vi "Take_C1_C2_Then_C1+C2.vi"(3 "Mode":T5, 5 "Traverse line In":T2 {"Row Duration (mins)" format="%#.1f"; "Row No" min=0; "Trace Gas Concentration (%)" min=0.0 format="%#.2f"; "Emission Rate (l/min)" format="%#.2f"; "Tunnel Speed" format="%#.2f"; "Start X" format="%#.2f"; "Start Y" format="%#.2f"; "Start Z" format="%#.2f"; "End X" format="%#.2f"; "End Y" format="%#.2f"; "End Z" format="%#.2f"; "Averaging time (min)" min=0.0 format="%#.1f"}) -> (0 "Error Message":string, 1 "Status":T1, 2 "Traverse line Out":T2 {"Row Duration (mins)" format="%#.1f"; "Row No" min=0; "Trace Gas Concentration (%)" min=0.0 format="%#.2f"; "Emission Rate (l/min)" format="%#.2f"; "Tunnel Speed" format="%#.2f"; "Start X" format="%#.2f"; "Start Y" format="%#.2f"; "Start Z" format="%#.2f"; "End X" format="%#.2f"; "End Y" format="%#.2f"; "End Z" format="%#.2f"; "Averaging time (min)" min=0.0 format="%#.1f"})   [LabVIEW 2010]
uses:
  Gen Trav/Traverse_cluster.ctl
  Gen Trav/Spacing.ctl
  Controls/Multi_run_mode.ctl
  Controls/User_Specific_mode.ctl
  Gen Trav/Multi_Run_Status.ctl
  Controls/Save_Data.ctl
  Controls/Setup.ctl
  Plug in sub vis/Extra_info.vi
  Globals/Meas_global.vi
panel:
  out "UA/Q 2":dbl
  out "UA/Q":dbl
  out "Source1 Ref?":bool
  out "Reference Position":dbl
  out "XY Graph":cluster{dbl[], dbl[]}(graph)
  out "Ch Values":string[](array[string])
  out "Ch Names":string[](array[string])
  # "X           Y            Z"
  # "Start"
  # "End"
  # "X           Y            Z"
  # "Start"
  # "End"
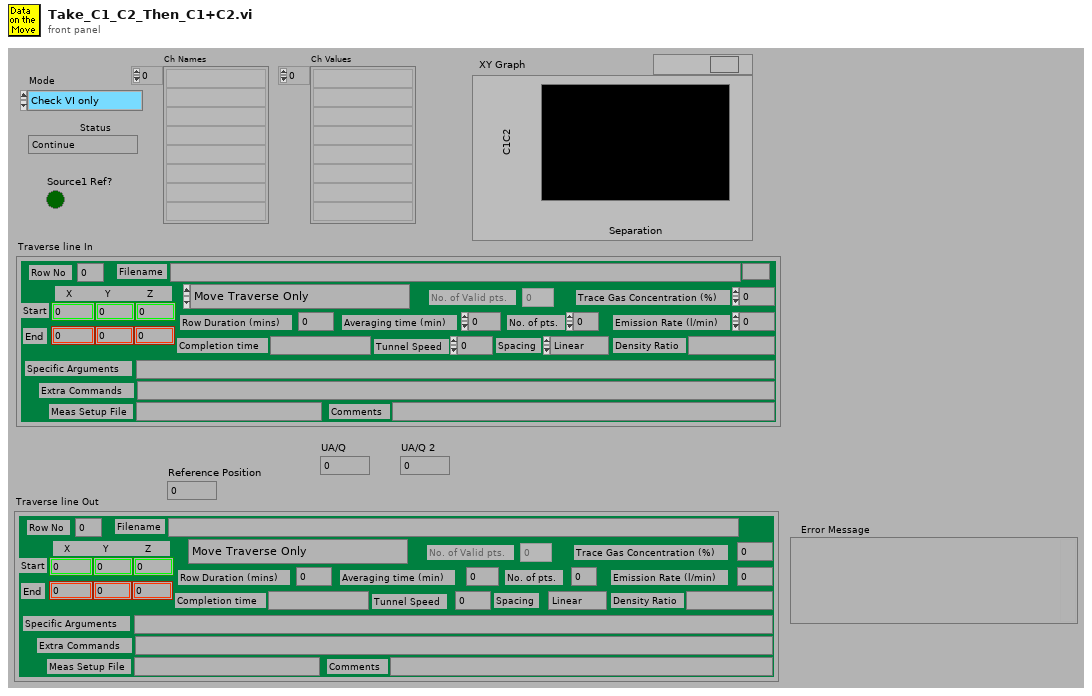
[diagram p1: front panel]
types:
  T1 = typedef "Multi_Run_Status.ctl" = enum16{"Continue", "Jump to Next Point", "Jump to Next Row", "Jump To Fall Back", "Terminate Run"}
  T2 = typedef "Traverse_cluster.ctl" = cluster{"Start X":dbl, "Start Y":dbl, "Start Z":dbl, "End X":dbl, "End Y":dbl, "End Z":dbl, "No. of pts.":i32, "Spacing":T3, "Filename":path, "Tunnel Speed":dbl, "Averaging time (min)":dbl, "Extra Commands":string, "Specific Arguments":string, "Emission Rate (l/min)":dbl, "Trace Gas Concentration (%)":dbl, "Density Ratio":string, "Comments":string, "Row No":i32, "Row Type Selector":T4, "Completion time":string, "Row Duration (mins)":dbl, "No. of Valid pts.":i32, "Meas Setup File":string}
  T3 = typedef "Spacing.ctl" = enum16{"Linear", "Log", "Gauss", "Specified", "N/A"}
  T4 = typedef "Multi_run_mode.ctl" = enum16{"Move Traverse Only", "Set Tunnel Speed Only", "Set Source Only", "Set Measurement Conditions", "Single Measurement", "Vertical Profile", "Lateral Profile", "Longitudinal Profile", "Explore Volume", "Multi-Axis Profile", "Auto Calibrate", "Meas Fast FID Bkgnd", "Check Beam Power", "Scanning Valve Measurement", "Run VI Named:", "Set ADAM Ch", "Wait (minutes)", "Send Message", "Synchronize With:", "Fall Back to this Row", "Turn Off Row Repeating", "Blank Row"}
  T5 = typedef "User_Specific_mode.ctl" = enum16{"Check VI only", "Run VI"}
  T6 = enum16{"Source 1 only", "Source 2 only", "Both Sources"}
  T7 = typedef "Save_Data.ctl" = enum16{"Save No Data", "Save Data"}
  T8 = typedef "Setup.ctl" = enum16{"Run Program", "Show Setup", "Save Current Setup", "Setup Front Panel"}
  T9 = typedef "Status_Cluster.ctl" = cluster{"Status":T1, "Error Type":string, "Error Description":string}
  T10 = typedef "Velocity_cluster.ctl" = cluster{"Name":string, "U":dbl, "u^2":dbl, "u^3/(u^2)^(1.5)":dbl, "u^4/(u^2)^2 -3":dbl, "% u'/U":dbl, "Mean % Err":dbl, "u^4":dbl}
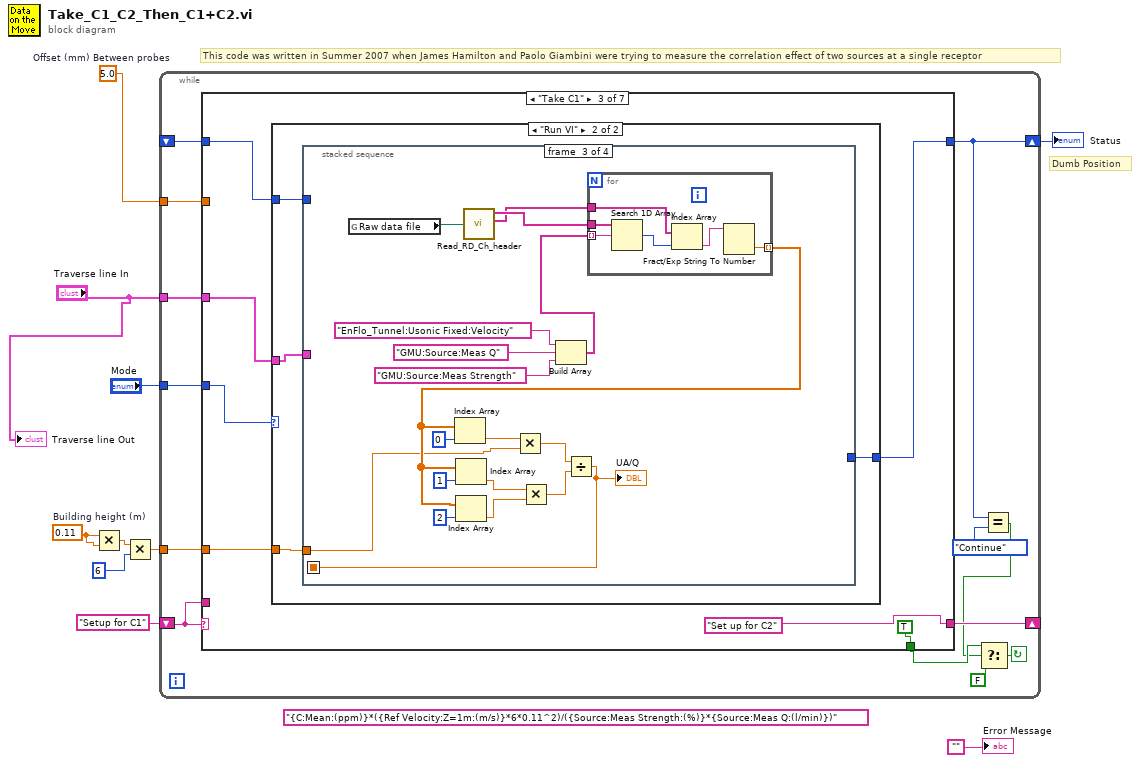
[diagram p0: block diagram]
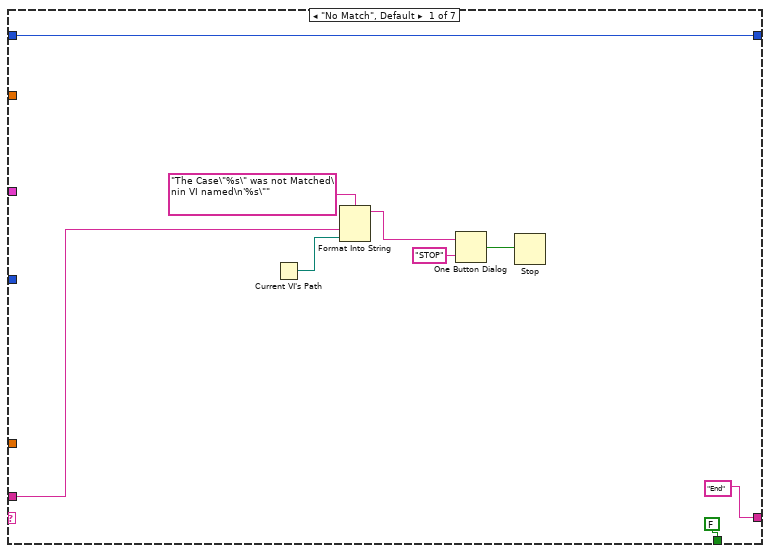
[diagram p2: hidden frame]
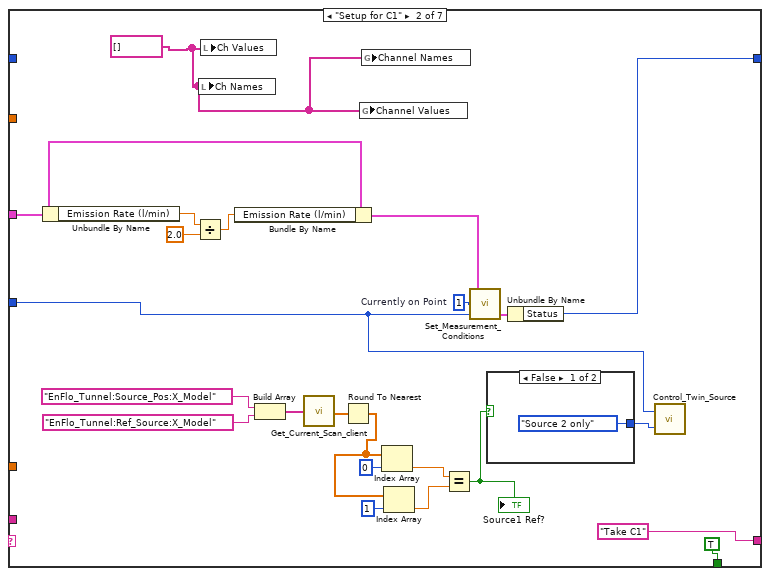
[diagram p3: hidden frame]
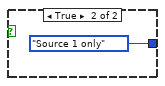
[diagram p4: hidden frame]
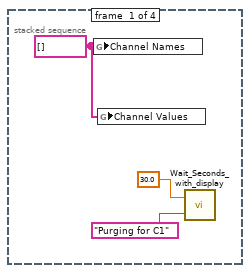
[diagram p6: hidden frame]
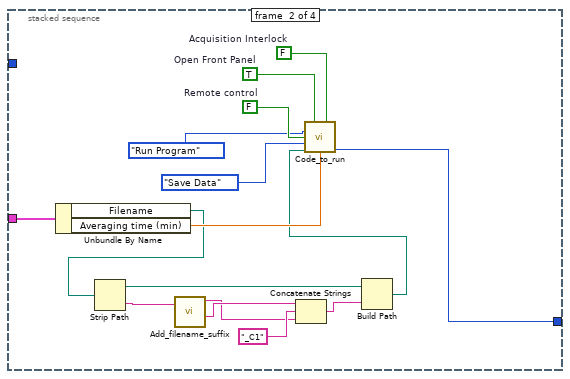
[diagram p7: hidden frame]
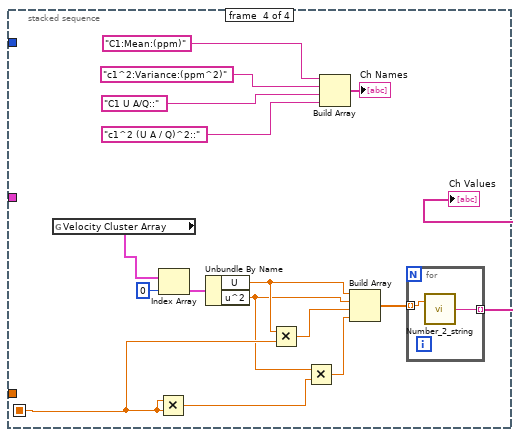
[diagram p8: hidden frame]
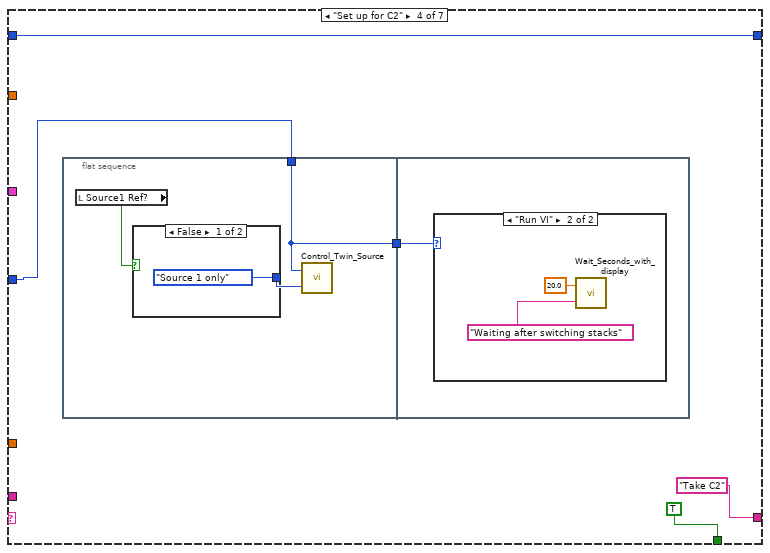
[diagram p9: hidden frame]
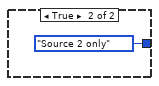
[diagram p10: hidden frame]
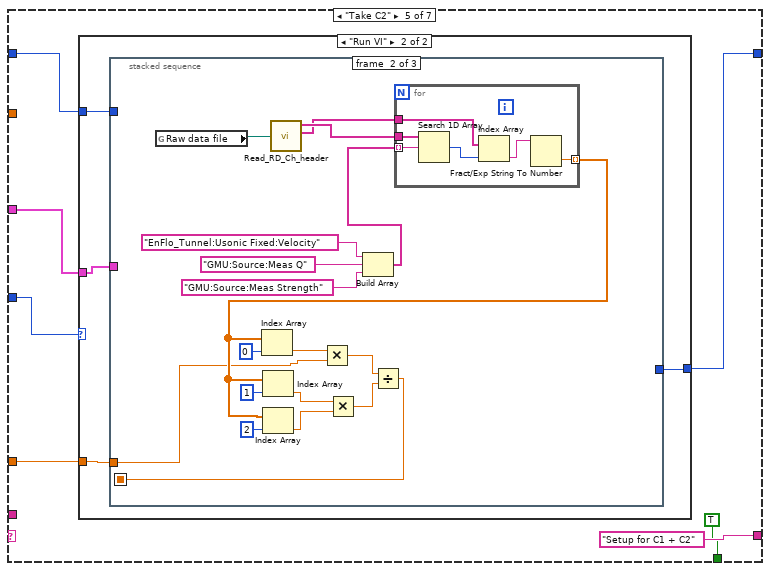
[diagram p12: hidden frame]
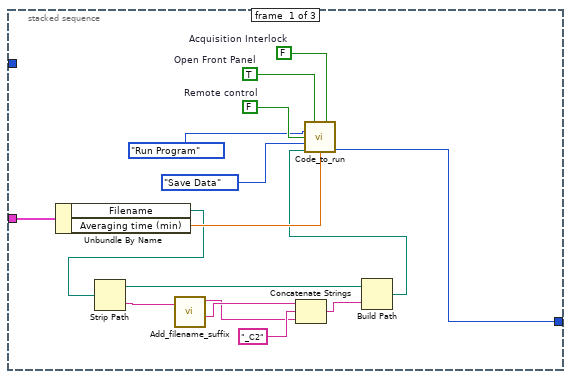
[diagram p14: hidden frame]
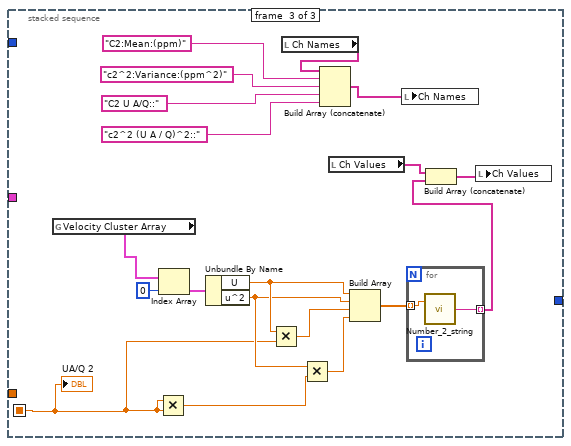
[diagram p15: hidden frame]
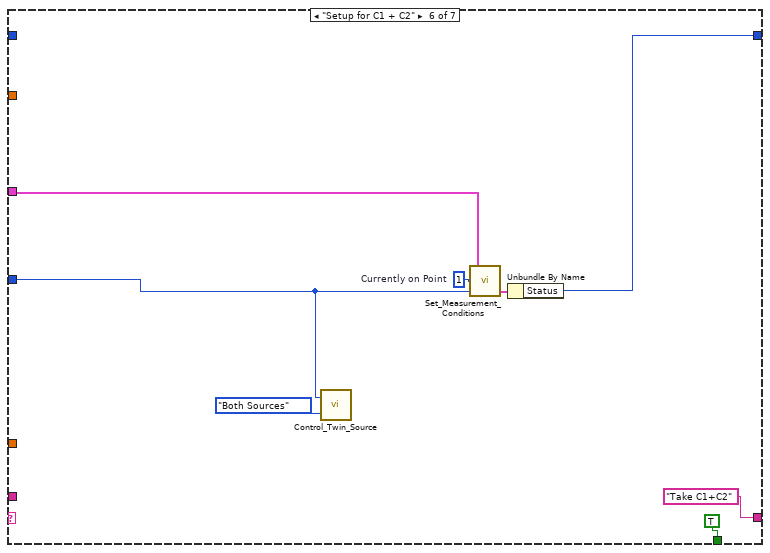
[diagram p16: hidden frame]
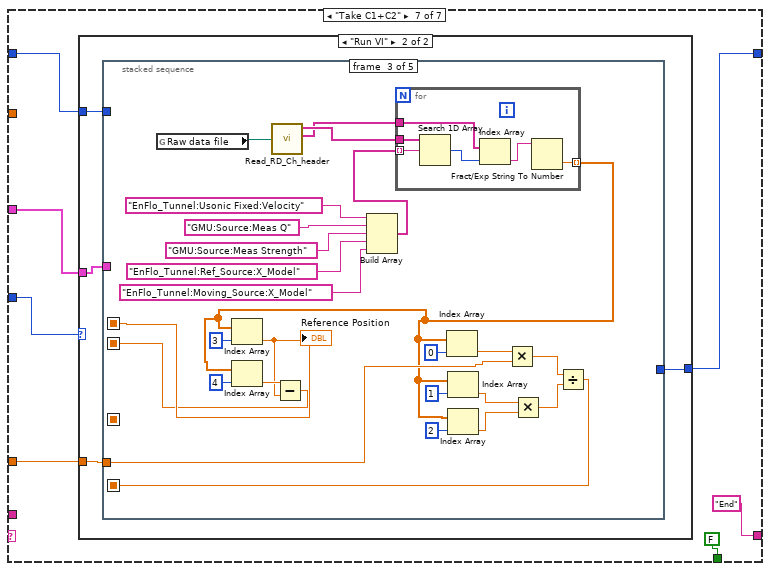
[diagram p17: hidden frame]
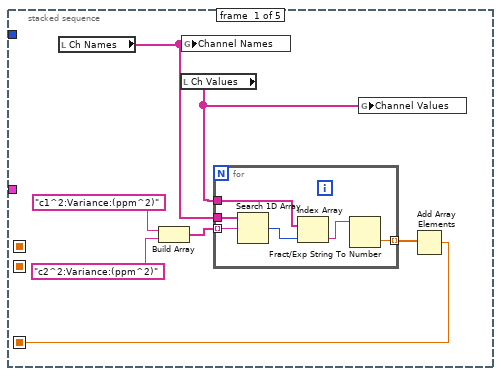
[diagram p19: hidden frame]
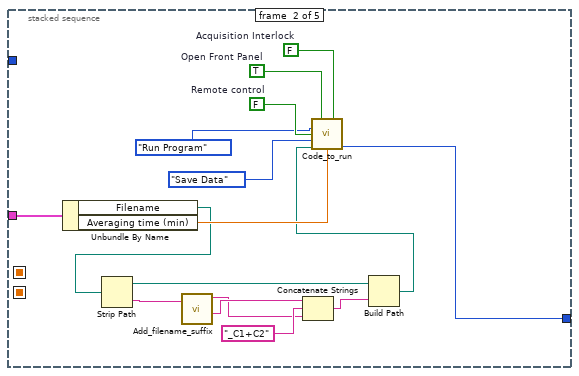
[diagram p20: hidden frame]
diagram:
  w5 = 0.11  # Building height (m)
  (unwired) "{C:Mean:(ppm)}*({Ref Velocity:Z=1m:(m/s)}*6*0.11^2)/({Source:Meas Strength:(%)}*{Source:Meas Q:(l/min)})"
  w7 = 5.0  # Offset (mm) Between probes
  # "This code was written in Summer 2007 when James Hamilton and Paolo Giambini were trying to measure the correlation effect of two sources at a single receptor"
  # "Dumb Position"
  n1 = Multiply(x=w5, y=w5) -> (x*y=w4:dbl)
  n2 = Multiply(x=w4, y=6) -> (x*y=w2:dbl)
  n3 = while {
    shift-left: _ -> [w20]
    shift-right: [w15] -> w8
    tunnel: "Traverse line In" -> [w22]
    tunnel: "Mode" -> [w23]
    shift-left: "Setup for C1" -> [w21]
    shift-right: [w19] -> _
    tunnel: w7 -> [w12]
    tunnel: w2 -> [w11]
    stop <- w13 continue-if-true
    n4 = case shown="\"Take C1\"" w21 {
      tunnel: w22 -> [_ w53 w63 _ w149 w221 w230]
      tunnel: w23 -> [_ w36 w64 w132 w150 w217 w231]
      tunnel: [FALSE ("Update Datum Powers?") TRUE ("Update Datum Powers?") TRUE ("Update Datum Powers?") TRUE ("Update Datum Powers?") TRUE ("Update Datum Powers?") TRUE ("Update Datum Powers?") FALSE ("Update Datum Powers?")] -> w18
      tunnel: ["End" "Take C1" "Set up for C2" "Take C2" "Setup for C1 + C2" "Take C1+C2" "End"] -> w19
      tunnel: w21 -> [w25 _ _ _ _ _ _]
      tunnel: w20 -> [w24 _ w61 w135 w147 _ w228]
      tunnel: [w24 w48 w58 w135 w144 w219 w225] -> w15
      tunnel: w12 -> [_ _ _ _ _ _ _]
      tunnel: w11 -> [_ _ w62 _ w148 _ w229]
      frame "No Match", Default {
        n5 = Current VI's Path() -> (path=w28:path)
        n6 = Format Into String(format string="The Case\"%s\" was not Matched\nin VI named\n'%s\"" ("Format String"), w25, w28) -> (resulting string=w31:string)  [unwired: 2 in, 1 out]
        n7 = One Button Dialog(message=w31, button name ("OK")="STOP") -> (true=w29:bool)
        n8 = Stop(stop? (T)=w29) -> ()
      }
      frame "Setup for C1" {
        w35 = string[] [] ("Ch Values")
        w54 = 1  # Currently on Point
        n9 = Unbundle By Name(w53) -> ("Emission Rate (l/min)"=w52:dbl)
        n10 = Divide(x=w52, y=2.0) -> (x/y=w50:dbl)
        n11 = local write "Ch Names"(w35) -> ()
        n12 = local write "Ch Values"(w35) -> ()
        n13 = Bundle By Name(cluster=w53, "Emission Rate (l/min)"=w50) -> (w49:T2)
        n14 = Build Array("EnFlo_Tunnel:Source_Pos:X_Model", "EnFlo_Tunnel:Ref_Source:X_Model" ("Channel Name")) -> (w43:string[])
        n15 = call "Get_Current_Scan_client.vi"("ADAM Ch Names"=w43) -> ("Numerical Values"=w34:dbl[])  [unwired: 3 out]
        n16 = Round To Nearest(number=w34) -> (nearest integer value=w33:dbl[])
        n17 = global write "Extra_info.vi" "Channel Values"(w35) -> ()
        n18 = global write "Extra_info.vi" "Channel Names"(w35) -> ()
        n19 = Index Array(array=w33, index=0) -> (element=w39:dbl)
        n20 = Index Array(array=w33, index=1) -> (element=w40:dbl)
        n21 = Equal?(x=w39, y=w40) -> (x = y?=w38:bool)
        "Source1 Ref?" <- w38
        n22 = call "Set_Measurement_Conditions.vi"("Simulate/Run"=w36, "Currently on Point"=w54, "Traverse line"=w49) -> ("Status Cluster"=w55:T9)  [unwired: 2 out]
        n23 = case shown="False" w38 {
          tunnel: [T6."Source 2 only" ("Mode") T6."Source 1 only" ("Mode")] -> w37
          frame False {
          }
          frame True {
          }
        }
        n24 = Unbundle By Name(w55) -> ("Status"=w48:T1)
        n25 = call "Control_Twin_Source.vi"("Control"=w37, "Mode"=w36) -> ()
      }
      frame "Take C1" {
        n26 = case shown="\"Run VI\"" w64 {
          tunnel: [w65 w69] -> w58
          tunnel: w63 -> [_ w68]
          tunnel: w62 -> [_ w67]
          tunnel: w61 -> [w65 w66]
          frame "Check VI only" {
          }
          frame "Run VI" {
            n27 = stacked-sequence {
              seq-local: [_ _ w89 _] -> [_ _ _ w119]
              tunnel: [_ w88 _ _] -> w69
              tunnel: w68 -> [_ w87 _ _]
              tunnel: w67 -> [_ _ w94 _]
              tunnel: w66 -> [_ _ _ _]
              frame #0 {
                w72 = string[] [] ("Channel Names")
                n28 = global write "Extra_info.vi" "Channel Names"(w72) -> ()
                n29 = global write "Extra_info.vi" "Channel Values"(w72) -> ()
                n30 = call "Wait_Seconds_with_display.vi"("Message"="Purging for C1", "Seconds to wait"=30.0) -> ()  [unwired: 2 out]
              }
              frame #1 {
                w83 = FALSE  # Acquisition Interlock
                w84 = TRUE  # Open Front Panel
                w86 = FALSE  # Remote control
                n31 = Unbundle By Name(w87) -> ("Filename"=w74:path, "Averaging time (min)"=w85:dbl)
                n32 = Strip Path(path=w74) -> (stripped path=w75:path, name=w80:string)
                n33 = call "Add_filename_suffix.vi"("Filename"=w80) -> ("Original Suffix"=w77:string, "Base name"=w79:string)  [unwired: 1 in, 2 out]
                n34 = Concatenate Strings(w79, "_C1" ("string"), w77) -> (w76:string)
                n35 = Build Path(base path=w75, name or relative path=w76) -> (appended path=w73:path)
                n36 = call "Code_to_run.vi"("Open Front Panel"=w84, "Acquisition Interlock"=w83, "setup"=Setup."Run Program", "Remote control"=w86, "File"=Save_Data."Save Data", "Results Filename"=w73, "Averaging time (min)"=w85) -> ("Status"=w88:T1)  [unwired: 4 in, 4 out]
              }
              frame #2 {
                n37 = global read "Meas_global.vi" "Raw data file"() -> (w105:path)
                n38 = call "Read_RD_Ch_header.vi"("Raw data file"=w105) -> ("Ch Name Out"=w103:string[], "Ch Values"=w102:string[])  [unwired: 2 out]
                n39 = Build Array("EnFlo_Tunnel:Usonic Fixed:Velocity", "GMU:Source:Meas Q", "GMU:Source:Meas Strength") -> (w104:string[])
                n40 = for {
                  tunnel: w103 -> [w112]
                  tunnel: w104 -> [w111] mode=indexing
                  tunnel: w102 -> [w109]
                  tunnel: [w107] -> w101 mode=indexing
                  n41 = Search 1D Array(1D array=w112, element=w111) -> (index of element=w110:i32)  [unwired: 1 out]
                  n42 = Index Array(array=w109, index=w110) -> (element=w108:string)
                  n43 = Fract/Exp String To Number(string=w108) -> (number=w107:dbl)  [unwired: 4 out]
                }
                n44 = Index Array(array=w101, index=0) -> (element=w95:dbl)
                n45 = Index Array(array=w101, index=1) -> (element=w93:dbl)
                n46 = Index Array(array=w101, index=2) -> (element=w92:dbl)
                n47 = Multiply(x=w95, y=w94) -> (x*y=w91:dbl)
                n48 = Multiply(x=w93, y=w92) -> (x*y=w90:dbl)
                n49 = Divide(x=w91, y=w90) -> (x/y=w89:dbl)
                "UA/Q" <- w89
              }
              frame #3 {
                n50 = global read "Meas_global.vi" "Velocity Cluster Array"() -> (w128:T10[])
                n51 = Multiply(x=w119, y=w119) -> (x*y=w115:dbl)
                n52 = Index Array(array=w128, index=0) -> (element=w126:T10)
                n53 = Unbundle By Name(w126) -> ("U"=w120:dbl, "u^2"=w117:dbl)
                n54 = Multiply(x=w120, y=w119) -> (x*y=w118:dbl)
                n55 = Multiply(x=w117, y=w115) -> (x*y=w116:dbl)
                n56 = Build Array("C1:Mean:(ppm)", "c1^2:Variance:(ppm^2)", "C1 U A/Q::", "c1^2 (U A / Q)^2::") -> (→"Ch Names":string[])
                n57 = Build Array(w120, w117, w118, w116) -> (w114:dbl[])
                n58 = for {
                  tunnel: w114 -> [w130] mode=indexing
                  tunnel: [w129] -> w113 mode=indexing
                  n59 = call "Number_2_string.vi"("number"=w130) -> ("String"=w129:string)  [unwired: 1 in]
                }
                "Ch Values" <- w113
              }
            }
          }
        }
      }
      frame "Set up for C2" {
        n60 = flat-sequence {
          tunnel: w132 -> [w136]
          tunnel: [w136] -> w131
          tunnel: w131 -> [w141]
          frame #0 {
            n61 = local read "Source1 Ref?"() -> (w137:bool)
            n62 = case shown="False" w137 {
              tunnel: [T6."Source 1 only" ("Mode") T6."Source 2 only" ("Mode")] -> w138
              frame False {
              }
              frame True {
              }
            }
            n63 = call "Control_Twin_Source.vi"("Control"=w138, "Mode"=w136) -> ()
          }
          frame #1 {
            n64 = case shown="\"Run VI\"" w141 {
              frame "Check VI only" {
              }
              frame "Run VI" {
                n65 = call "Wait_Seconds_with_display.vi"("Message"="Waiting after switching stacks", "Seconds to wait"=20.0) -> ()  [unwired: 2 out]
              }
            }
          }
        }
      }
      frame "Take C2" {
        n66 = case shown="\"Run VI\"" w150 {
          tunnel: [w151 w155] -> w144
          tunnel: w149 -> [_ w154]
          tunnel: w148 -> [_ w153]
          tunnel: w147 -> [w151 w152]
          frame "Check VI only" {
          }
          frame "Run VI" {
            n67 = stacked-sequence {
              seq-local: [_ w172 _] -> [_ _ w196]
              tunnel: [w171 _ _] -> w155
              tunnel: w154 -> [w170 _ _]
              tunnel: w153 -> [_ w177 _]
              tunnel: w152 -> [_ _ _]
              frame #0 {
                w166 = FALSE  # Acquisition Interlock
                w167 = TRUE  # Open Front Panel
                w169 = FALSE  # Remote control
                n68 = Unbundle By Name(w170) -> ("Filename"=w157:path, "Averaging time (min)"=w168:dbl)
                n69 = Strip Path(path=w157) -> (stripped path=w158:path, name=w163:string)
                n70 = call "Add_filename_suffix.vi"("Filename"=w163) -> ("Original Suffix"=w160:string, "Base name"=w162:string)  [unwired: 1 in, 2 out]
                n71 = Concatenate Strings(w162, "_C2" ("string"), w160) -> (w159:string)
                n72 = Build Path(base path=w158, name or relative path=w159) -> (appended path=w156:path)
                n73 = call "Code_to_run.vi"("Open Front Panel"=w167, "Acquisition Interlock"=w166, "setup"=Setup."Run Program", "Remote control"=w169, "File"=Save_Data."Save Data", "Results Filename"=w156, "Averaging time (min)"=w168) -> ("Status"=w171:T1)  [unwired: 4 in, 4 out]
              }
              frame #1 {
                n74 = global read "Meas_global.vi" "Raw data file"() -> (w188:path)
                n75 = call "Read_RD_Ch_header.vi"("Raw data file"=w188) -> ("Ch Name Out"=w186:string[], "Ch Values"=w185:string[])  [unwired: 2 out]
                n76 = Build Array("EnFlo_Tunnel:Usonic Fixed:Velocity", "GMU:Source:Meas Q", "GMU:Source:Meas Strength") -> (w187:string[])
                n77 = for {
                  tunnel: w186 -> [w195]
                  tunnel: w187 -> [w194] mode=indexing
                  tunnel: w185 -> [w192]
                  tunnel: [w190] -> w184 mode=indexing
                  n78 = Search 1D Array(1D array=w195, element=w194) -> (index of element=w193:i32)  [unwired: 1 out]
                  n79 = Index Array(array=w192, index=w193) -> (element=w191:string)
                  n80 = Fract/Exp String To Number(string=w191) -> (number=w190:dbl)  [unwired: 4 out]
                }
                n81 = Index Array(array=w184, index=0) -> (element=w178:dbl)
                n82 = Index Array(array=w184, index=1) -> (element=w176:dbl)
                n83 = Index Array(array=w184, index=2) -> (element=w175:dbl)
                n84 = Multiply(x=w178, y=w177) -> (x*y=w174:dbl)
                n85 = Multiply(x=w176, y=w175) -> (x*y=w173:dbl)
                n86 = Divide(x=w174, y=w173) -> (x/y=w172:dbl)
              }
              frame #2 {
                n87 = global read "Meas_global.vi" "Velocity Cluster Array"() -> (w214:T10[])
                n88 = Multiply(x=w196, y=w196) -> (x*y=w203:dbl)
                n89 = Index Array(array=w214, index=0) -> (element=w212:T10)
                n90 = Unbundle By Name(w212) -> ("U"=w207:dbl, "u^2"=w205:dbl)
                n91 = Multiply(x=w207, y=w196) -> (x*y=w206:dbl)
                n92 = local read "Ch Names"() -> (w201:string[])
                n93 = Multiply(x=w205, y=w203) -> (x*y=w204:dbl)
                n94 = Build Array (concatenate)(w201, "C2:Mean:(ppm)", "c2^2:Variance:(ppm^2)", "C2 U A/Q::", "c2^2 (U A / Q)^2::") -> (w200:string[])
                n95 = local read "Ch Values"() -> (w199:string[])
                n96 = Build Array(w207, w205, w206, w204) -> (w202:dbl[])
                n97 = local write "Ch Names"(w200) -> ()
                n98 = for {
                  tunnel: w202 -> [w216] mode=indexing
                  tunnel: [w215] -> w198 mode=indexing
                  n99 = call "Number_2_string.vi"("number"=w216) -> ("String"=w215:string)  [unwired: 1 in]
                }
                n100 = Build Array (concatenate)(w199, w198) -> (w197:string[])
                n101 = local write "Ch Values"(w197) -> ()
                "UA/Q 2" <- w196
              }
            }
          }
        }
      }
      frame "Setup for C1 + C2" {
        w223 = 1  # Currently on Point
        n102 = call "Control_Twin_Source.vi"("Control"=T6."Both Sources" ("Mode"), "Mode"=w217) -> ()
        n103 = call "Set_Measurement_Conditions.vi"("Simulate/Run"=w217, "Currently on Point"=w223, "Traverse line"=w221) -> ("Status Cluster"=w224:T9)  [unwired: 2 out]
        n104 = Unbundle By Name(w224) -> ("Status"=w219:T1)
      }
      frame "Take C1+C2" {
        n105 = case shown="\"Run VI\"" w231 {
          tunnel: [w232 w236] -> w225
          tunnel: w230 -> [_ w235]
          tunnel: w229 -> [_ w234]
          tunnel: w228 -> [w232 w233]
          frame "Check VI only" {
          }
          frame "Run VI" {
            n106 = stacked-sequence {
              seq-local: [_ _ w274 _ _] -> [_ _ _ _ _]
              seq-local: [w237 _ _ _ _] -> [_ _ _ w306 _]
              seq-local: [_ _ w267 _ _] -> [_ _ _ w303 _]
              seq-local: [_ _ w266 _ _] -> [_ _ _ w302 _]
              tunnel: [_ w265 _ _ _] -> w236
              tunnel: w235 -> [_ w264 _ _ _]
              tunnel: w234 -> [_ _ w275 _ _]
              tunnel: w233 -> [_ _ _ _ _]
              frame #0 {
                n107 = local read "Ch Names"() -> (w240:string[])
                n108 = Build Array("c1^2:Variance:(ppm^2)", "c2^2:Variance:(ppm^2)") -> (w241:string[])
                n109 = local read "Ch Values"() -> (w239:string[])
                n110 = global write "Extra_info.vi" "Channel Names"(w240) -> ()
                n111 = for {
                  tunnel: w240 -> [w249]
                  tunnel: w241 -> [w248] mode=indexing
                  tunnel: w239 -> [w246]
                  tunnel: [w244] -> w238 mode=indexing
                  n112 = Search 1D Array(1D array=w249, element=w248) -> (index of element=w247:i32)  [unwired: 1 out]
                  n113 = Index Array(array=w246, index=w247) -> (element=w245:string)
                  n114 = Fract/Exp String To Number(string=w245) -> (number=w244:dbl)  [unwired: 4 out]
                }
                n115 = global write "Extra_info.vi" "Channel Values"(w239) -> ()
                n116 = Add Array Elements(numeric array=w238) -> (sum=w237:dbl)
              }
              frame #1 {
                w260 = FALSE  # Acquisition Interlock
                w261 = TRUE  # Open Front Panel
                w263 = FALSE  # Remote control
                n117 = Unbundle By Name(w264) -> ("Filename"=w251:path, "Averaging time (min)"=w262:dbl)
                n118 = Strip Path(path=w251) -> (stripped path=w252:path, name=w257:string)
                n119 = call "Add_filename_suffix.vi"("Filename"=w257) -> ("Original Suffix"=w254:string, "Base name"=w256:string)  [unwired: 1 in, 2 out]
                n120 = Concatenate Strings(w256, "_C1+C2" ("string"), w254) -> (w253:string)
                n121 = Build Path(base path=w252, name or relative path=w253) -> (appended path=w250:path)
                n122 = call "Code_to_run.vi"("Open Front Panel"=w261, "Acquisition Interlock"=w260, "setup"=Setup."Run Program", "Remote control"=w263, "File"=Save_Data."Save Data", "Results Filename"=w250, "Averaging time (min)"=w262) -> ("Status"=w265:T1)  [unwired: 4 in, 4 out]
              }
              frame #2 {
                n123 = global read "Meas_global.vi" "Raw data file"() -> (w289:path)
                n124 = call "Read_RD_Ch_header.vi"("Raw data file"=w289) -> ("Ch Name Out"=w287:string[], "Ch Values"=w286:string[])  [unwired: 2 out]
                n125 = Build Array("EnFlo_Tunnel:Usonic Fixed:Velocity", "GMU:Source:Meas Q", "GMU:Source:Meas Strength", "EnFlo_Tunnel:Ref_Source:X_Model" ("Channel Name"), "EnFlo_Tunnel:Moving_Source:X_Model" ("Channel Name")) -> (w288:string[])
                n126 = for {
                  tunnel: w287 -> [w296]
                  tunnel: w288 -> [w295] mode=indexing
                  tunnel: w286 -> [w293]
                  tunnel: [w291] -> w269 mode=indexing
                  n127 = Search 1D Array(1D array=w296, element=w295) -> (index of element=w294:i32)  [unwired: 1 out]
                  n128 = Index Array(array=w293, index=w294) -> (element=w292:string)
                  n129 = Fract/Exp String To Number(string=w292) -> (number=w291:dbl)  [unwired: 4 out]
                }
                n130 = Index Array(array=w269, index=3) -> (element=w267:dbl)
                "Reference Position" <- w267
                n131 = Index Array(array=w269, index=4) -> (element=w268:dbl)
                n132 = Subtract(x=w268, y=w267) -> (x-y=w266:dbl)
                n133 = Index Array(array=w269, index=0) -> (element=w280:dbl)
                n134 = Index Array(array=w269, index=1) -> (element=w279:dbl)
                n135 = Index Array(array=w269, index=2) -> (element=w278:dbl)
                n136 = Multiply(x=w280, y=w275) -> (x*y=w277:dbl)
                n137 = Multiply(x=w279, y=w278) -> (x*y=w276:dbl)
                n138 = Divide(x=w277, y=w276) -> (x/y=w274:dbl)
              }
              frame #3 {
                # "(C1+C2)^2 = C1^2  + C2^2  + 2C1C2\nTherefore\nC1C2= ((C1+C2)^2  -C1^2  - C2^2)/2"
                n139 = global read "Meas_global.vi" "Velocity Cluster Array"() -> (w309:T10[])
                n140 = Index Array(array=w309, index=0) -> (element=w307:T10)
                n141 = Unbundle By Name(w307) -> ("u^2"=w297:dbl)
                n142 = Subtract(x=w297, y=w306) -> (x-y=w305:dbl)
                n143 = Divide(x=w305, y=2.0) -> (x/y=w301:dbl)
                n144 = while {
                  shift-right: [w318] -> _
                  shift-left: _ -> [w319]
                  tunnel: w303 -> [w318]
                  shift-right: [w311] -> w300
                  shift-left: _ -> [w316]
                  shift-right: [w312] -> w299
                  shift-left: _ -> [w315]
                  tunnel: w302 -> [w314]
                  tunnel: w301 -> [w313]
                  stop <- TRUE stop-if-true
                  n145 = Equal?(x=w319, y=w318) -> (x = y?=w317:bool)
                  n146 = case shown="False" w317 {
                    tunnel: w316 -> [_ w329]
                    tunnel: w315 -> [_ w328]
                    tunnel: w314 -> [w322 w327]
                    tunnel: w313 -> [w323 w326]
                    tunnel: [w320 w325] -> w312
                    tunnel: [w321 w324] -> w311
                    frame False {
                      n147 = Build Array(w322) -> (w321:dbl[])
                      n148 = Build Array(w323) -> (w320:dbl[])
                    }
                    frame True {
                      n149 = Build Array (concatenate)(w329, w327) -> (w324:dbl[])
                      n150 = Build Array (concatenate)(w328, w326) -> (w325:dbl[])
                    }
                  }
                }
                n151 = Bundle(w300, w299) -> (→"XY Graph":cluster{dbl[], dbl[]})  [unwired: 1 out]
              }
              frame #4 {
                w330 = string[] [] ("Ch Values")
                n152 = local write "Ch Names"(w330) -> ()
                n153 = local write "Ch Values"(w330) -> ()
                n154 = global write "Extra_info.vi" "Channel Values"(w330) -> ()
                n155 = global write "Extra_info.vi" "Channel Names"(w330) -> ()
              }
            }
          }
        }
      }
    }
    n156 = Equal?(x=w15, y=Multi_Run_Status."Continue" ("Status")) -> (x = y?=w17:bool)
    n157 = Select(t=w18, s=w17, f=FALSE) -> (s? t:f=w13:bool)
  }
  "Status" <- w8
  "Error Message" <- ""
  "Traverse line Out" <- "Traverse line In"
